vi "Read_indicator.vi"(8 "error in":errorcluster, 10 "Idicator_label":string, 11 "VI Refnum":refnum<vi>) -> (0 "error out":errorcluster, 2 "data":variant, 3 "ref out":refnum<vi>)   [LabVIEW 2020]
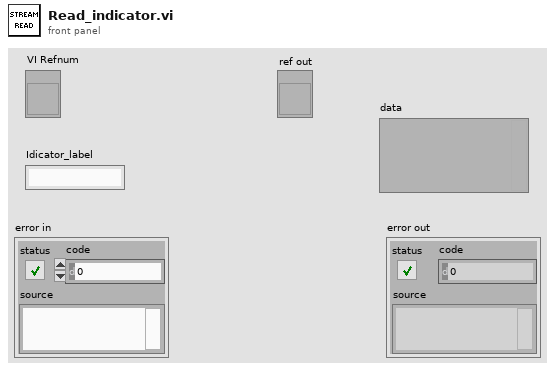
[diagram p1: front panel]
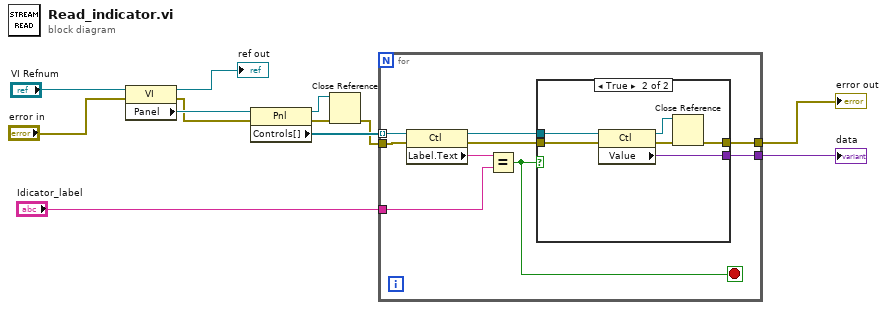
[diagram p0: block diagram]
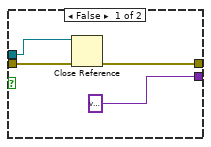
[diagram p2: hidden frame]
diagram:
  n1 = property class="VI"(reference="VI Refnum", error in="error in") -> (reference out=→"ref out":refnum<vi>, error out=w2:errorcluster, "Panel"=w11:refnum<vi>)
  n2 = property class="Pnl"(reference=w11, error in=w2) -> (reference out=w8:refnum<vi>, error out=w9:errorcluster, "Controls[]"=w10:refnum<vi>[])
  n3 = Close Reference(reference=w8, error in (no error)=w9) -> (error out=w6:errorcluster)
  n4 = for {
    tunnel: w10 -> [w21] mode=indexing
    tunnel: "Idicator_label" -> [w19]
    tunnel: w6 -> [w18]
    tunnel: [w14] -> w4
    tunnel: [w13] -> w3
    stop <- w17 stop-if-true
    n5 = property class="Ctl"(reference=w21, error in=w18) -> (reference out=w16:refnum<vi>, error out=w15:errorcluster, "Label.Text"=w20:string)
    n6 = Equal?(x=w20, y=w19) -> (x = y?=w17:bool)
    n7 = case shown="True" w17 {
      tunnel: w16 -> [w23 w31]
      tunnel: w15 -> [w25 w30]
      tunnel: [variant ("Value") w29] -> w14
      tunnel: [w24 w27] -> w13
      frame False {
        n8 = Close Reference(reference=w23, error in (no error)=w25) -> (error out=w24:errorcluster)
      }
      frame True {
        n9 = property class="Ctl"(reference=w31, error in=w30) -> (reference out=w26:refnum<vi>, error out=w28:errorcluster, "Value"=w29:variant)
        n10 = Close Reference(reference=w26, error in (no error)=w28) -> (error out=w27:errorcluster)
      }
    }
  }
  "error out" <- w3
  "data" <- w4
